vi "AES ECU Event Measurement - All Measurements.vi"(6 "Cycles to Filter":u16, 8 "Using Cycle Angle":bool, 10 "Digital Input Pulse":bool, 11 "Crank or Cyle Angle":fxp<+,61,10>) -> (0 "End Angle (degrees)":fxp<+,61,10> format="%.55g", 1 "Start Angle (degrees)":fxp<+,61,10> format="%.55g", 2 "Angle Duration (degrees)":fxp<+/-,62,11> format="%.55g", 3 "Time Duration (clock ticks)":u32)   [LabVIEW 2010, in "AES.lvlib" / "AES FPGA.lvlib"]
doc: "This IP inputs the fuel injector or ignition coil digital signals from an ECU and determines the Start Angle, End Angle, Angle Duration, and Time Duration of the pulses for those signals. This IP allows you to input either the crank (0-360) or cycle (0-720) angles. Set true on the Using Cycle Angle input if you are using the cycle angle. \n\nA \"Cycles to Filter\" input is also accepted in order to filter the digital inputs for a specified number of SCTL iterations. This is necessary since ECUs often output very noisy signals, and we need to filter it to get accurate calculations on the Start and End Angles."
uses:
  AES FPGA.lvlib
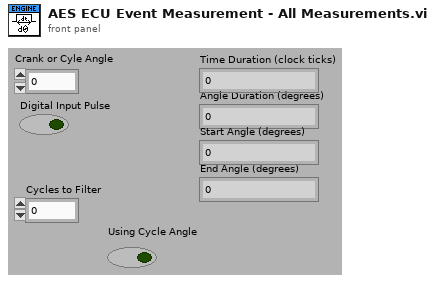
[diagram p1: front panel]
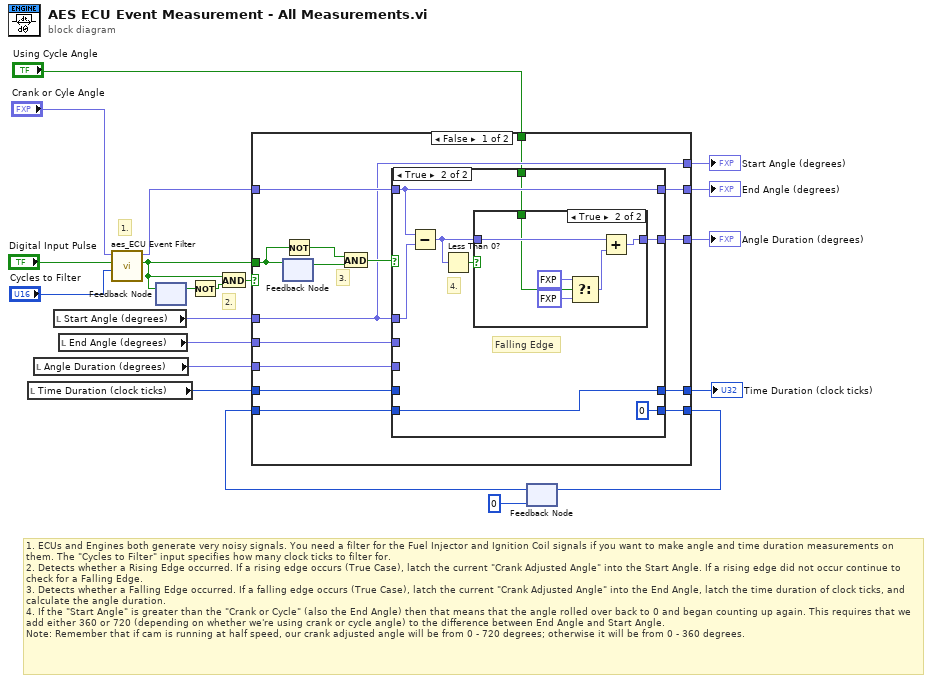
[diagram p0: block diagram]
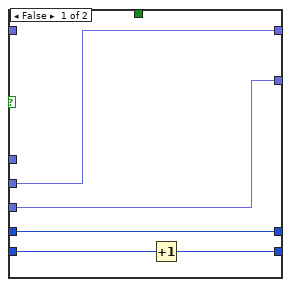
[diagram p2: hidden frame]
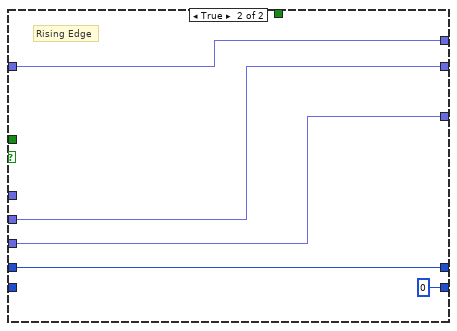
[diagram p4: hidden frame]
diagram:
  # "2."
  # "1. ECUs and Engines both generate very noisy signals. You need a filter for the Fuel Injector and Ignition Coil signals if you want to make angle and time duration measurements on them. The \"Cycles to Filter\" input specifies how many clock ticks to filter for.\n2. Detects whether a Rising Edge occurred. If a rising edge occurs (True Case), latch the current \"Crank Adjusted Angle\" into the Start Angle. If a rising edge did not occur continue to check for a Falling Edge.\n3. Detects whether a Falling Edge occurred. If a falling edge occurs (True Case), latch the current \"Crank Adjusted Angle\" into the End Angle, latch the time duration of clock ticks, and calculate the angle duration.\n4. If the \"Start Angle\" is greater than the \"Crank or Cycle\" (also the End Angle) then that means that the angle rolled over back to 0 and began counting up again. This requires that we add either 360 or 720 (depending on whether we're using crank or cycle angle) to the difference between End Angle and Start Angle.\nNote: Remember that if cam is running at half speed, our crank adjusted angle will be from 0 - 720 degrees; otherwise it will be from 0 - 360 degrees."
  # "1."
  n1 = local read "Time Duration (clock ticks)"() -> (w10:u32)
  n2 = local read "Angle Duration (degrees)"() -> (w3:fxp<+/-,62,11>)
  n3 = local read "Start Angle (degrees)"() -> (w12:fxp<+,61,10>)
  n4 = local read "End Angle (degrees)"() -> (w11:fxp<+,61,10>)
  n5 = call "aes_ECU Event Filter.vi"("Cycles to Filter"="Cycles to Filter", "Input Signal"="Digital Input Pulse", "Input Angle (degrees)"="Crank or Cyle Angle") -> ("Output Filtered Signal"=w5:bool, "Transitioned Angle"=w6:fxp<+,61,10>)  [unwired: 7 in]
  n6 = feedback-in #1(w5) -> ()
  n7 = feedback #1() -> (w20:bool)  [unwired: 1 out]
  n8 = Not(x=w20) -> (.not. x?=w19:bool)
  n9 = And(x=w5, y=w19) -> (x .and. y?=w15:bool)
  n10 = feedback #2(u32 0) -> (w8:u32)
  n11 = case shown="False" w15 {
    tunnel: w12 -> [w22 _]
    tunnel: w6 -> [w35 w60]
    tunnel: w5 -> [w31 _]
    tunnel: [w22 w60] -> w18
    tunnel: [w30 w56] -> w17
    tunnel: w3 -> [w29 w56]
    tunnel: [w28 w57] -> w16
    tunnel: w11 -> [w27 w57]
    tunnel: [w26 w59] -> w14
    tunnel: w10 -> [w25 w59]
    tunnel: [w24 u32 0] -> w9
    tunnel: w8 -> [w23 _]
    tunnel: "Using Cycle Angle" -> [w21 _]
    frame False {
      # "3."
      n12 = feedback-in #3(w31) -> ()
      n13 = feedback #3() -> (w33:bool)  [unwired: 1 out]
      n14 = Not(x=w31) -> (.not. x?=w32:bool)
      n15 = And(x=w32, y=w33) -> (x .and. y?=w34:bool)
      n16 = case shown="True" w34 {
        tunnel: w35 -> [_ w44]
        tunnel: w22 -> [_ w48]
        tunnel: [w36 w45] -> w30
        tunnel: w29 -> [w36 _]
        tunnel: [w37 w44] -> w28
        tunnel: w27 -> [w37 _]
        tunnel: [w40 w43] -> w26
        tunnel: w25 -> [w40 _]
        tunnel: [w39 u32 0] -> w24
        tunnel: w23 -> [w38 w43]
        tunnel: w21 -> [_ w41]
        frame False {
          n17 = Increment(x=w38) -> (x+1=w39:u32)
        }
        frame True {
          # "4."
          # "Falling Edge"
          n18 = Subtract(x=w44, y=w48) -> (x-y=w46:fxp<+/-,62,11>)
          n19 = Less Than 0?(x=w46) -> (x < 0?=w47:bool)
          n20 = case shown="True" w47 {
            tunnel: w46 -> [w49 w55]
            tunnel: [w49 w54] -> w45
            tunnel: w41 -> [_ w50]
            frame False {
            }
            frame True {
              n21 = Select(t=fxp<+,7,10> 720.0 ("y"), s=w50, f=fxp<+,6,9> 360.0 ("y")) -> (s? t:f=w51:fxp<+,7,10>)
              n22 = Add(x=w55, y=w51) -> (x+y=w54:fxp<+/-,62,11>)
            }
          }
        }
      }
    }
    frame True {
      # "Rising Edge"
    }
  }
  "Start Angle (degrees)" <- w18
  "Angle Duration (degrees)" <- w17
  "End Angle (degrees)" <- w16
  "Time Duration (clock ticks)" <- w14
  n23 = feedback-in #2(w9) -> ()
